vi "Initiate Voltage Sweep.vi"(8 "error in (no error)":errorcluster, 11 "VISA resource name":refnum<visa-resource-name>) -> (0 "error out":errorcluster, 3 "VISA resource name out":refnum<visa-resource-name>)   [LabVIEW 2020, in "Keithley 648X Series.lvlib"]
doc: "This low-level VI places the voltage source in operate and begins sweep operation with the next trigger. \n\n<B>Notes:</B> \n1) Use this VI only with other low-level VIs. The high-level VIs automatically incorporate this functionality. This VI does not check the instrument status. If you want to check the instrument status, call the <B>Error Query</B> VI at the conclusion of the sequence.\n2) <b>This VI is only valid for the model 6487</b>."
uses:
  <instrlib>/Keithley 648X Series/Keithley 648X Series.lvlib
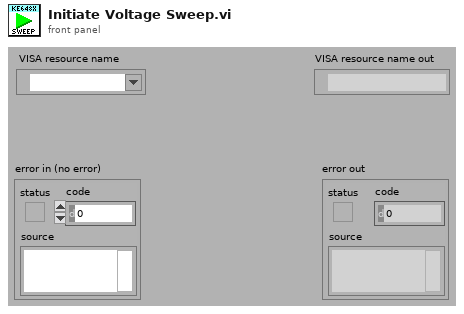
[diagram p1: front panel]
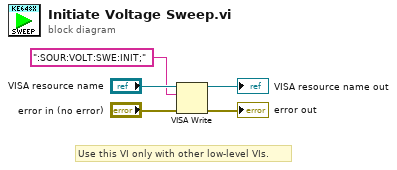
[diagram p0: block diagram]
diagram:
  # "Use this VI only with other low-level VIs."
  n1 = VISA Write(VISA resource name="VISA resource name", write buffer=":SOUR:VOLT:SWE:INIT;" ("Initiate"), error in (no error)="error in (no error)") -> (VISA resource name out=→"VISA resource name out":refnum<visa-resource-name>, error out=→"error out":errorcluster)  [unwired: 1 out]
